vi "Configure Fail Stop.vi"(0 "VISA resource name":refnum<visa-resource-name>, 7 "Fail Stop On/OFF (F:Off)":bool, 11 "error in (no error)":errorcluster) -> (4 "VISA resource name out":refnum<visa-resource-name>, 15 "error out":errorcluster)   [LabVIEW 2020, in "eec EST 300.lvlib"]
doc: "SF {1|0}\nSets the Fail Stop function ON or OFF for the active setup file loaded into RAM.\n\n1 setsthe Fail Stop = ON\n0 sets the Fail Stop = OFF"
uses:
  <instrlib>/eec EST 300/eec EST 300.lvlib
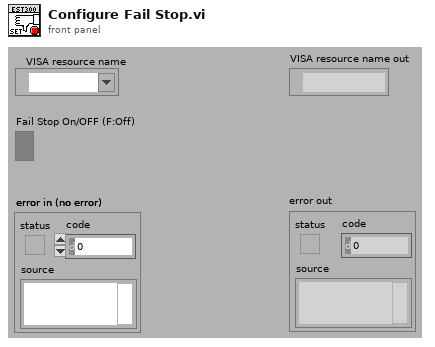
[diagram p1: front panel]
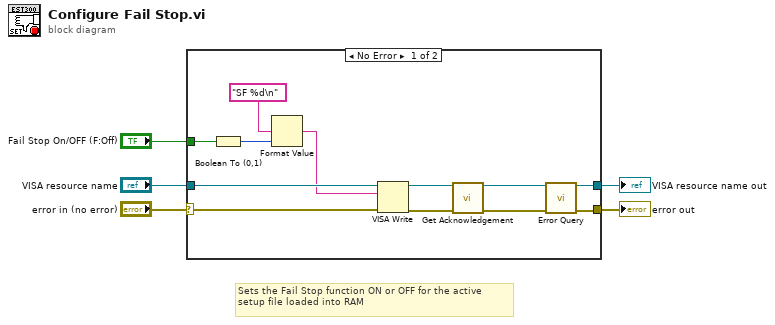
[diagram p0: block diagram]
diagram:
  # "Sets the Fail Stop function ON or OFF for the active setup file loaded into RAM"
  n1 = case shown="No Error" "error in (no error)" {
    selector: "error in (no error)" -> [w14 w19]
    tunnel: [w15 w19] -> w4
    tunnel: [w16 w18] -> w2
    tunnel: "VISA resource name" -> [w17 w18]
    tunnel: "Fail Stop On/OFF (F:Off)" -> [w13 _]
    frame No Error {
      n2 = Boolean To (0,1)(Boolean=w13) -> (0, 1=w6:i16)
      n3 = Format Value(format string="SF %d\n", value (0)=w6) -> (output string=w11:string)  [unwired: 1 in]
      n4 = VISA Write(VISA resource name=w17, write buffer=w11, error in (no error)=w14) -> (VISA resource name out=w8:refnum<visa-resource-name>, error out=w7:errorcluster)  [unwired: 1 out]
      n5 = call <instrlib>:"Get Acknowledgement.vi"("VISA resource name"=w8, "error in (no error)"=w7) -> ("VISA resource name out"=w10:refnum<visa-resource-name>, "error out"=w9:errorcluster)  [unwired: 12 in]
      n6 = call <instrlib>:"Error Query.vi"("VISA resource name"=w10, "error in (no error)"=w9) -> ("VISA resource name out"=w16:refnum<visa-resource-name>, "error out"=w15:errorcluster)  [unwired: 10 in, 2 out]
    }
    frame Error {
    }
  }
  "error out" <- w4
  "VISA resource name out" <- w2
